vi "GetFileVersion_DotNet.vi"(8 "error in (no error)":errorcluster, 11 "Exe Path":path) -> (0 "error out":errorcluster, 2 "File Info Out":T1, 3 "Exe Path Out":path)   [LabVIEW 2015]
doc: "This VI can obtain information about an existing executable, such as its version, product name, and so on, or it can be called as a subVI from a VI that will be built into an executable to obtain information about that executable.\n\nTo obtain version information about an existing executable, enter a path to an executable into Exe Path and run the Vi.\n\nCall this VI as a subVI from a VI that you will build into an executable and leave the path input unwired to obtain the version information about the built executable."
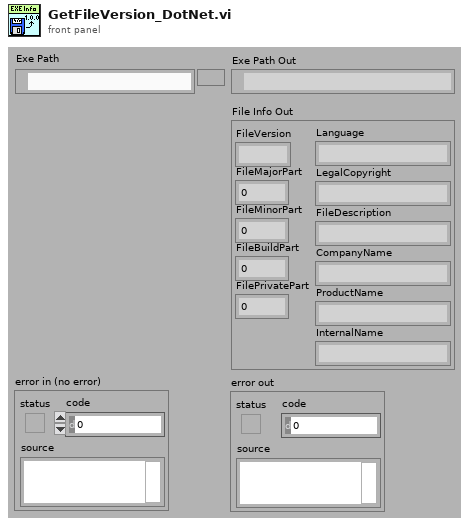
[diagram p1: front panel]
types:
  T1 = cluster{"FileVersion":string, "FileMajorPart":i32, "FileMinorPart":i32, "FileBuildPart":i32, "FilePrivatePart":i32, "Language":string, "LegalCopyright":string, "FileDescription":string, "CompanyName":string, "ProductName":string, "InternalName":string}
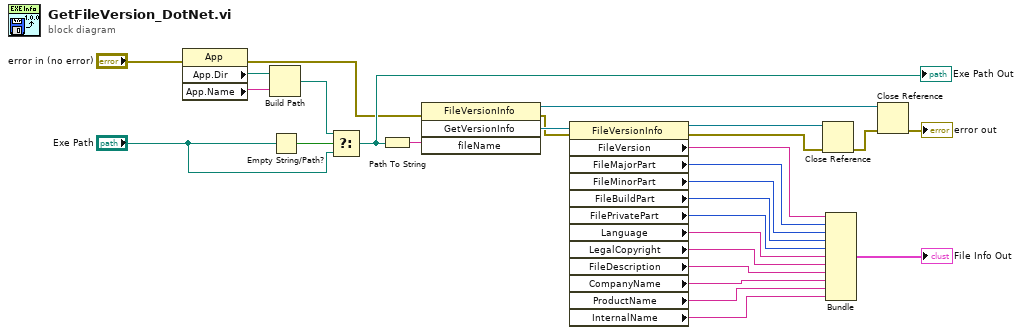
[diagram p0: block diagram]
diagram:
  n1 = property class="App"(error in="error in (no error)") -> (error out=w14:errorcluster, "App.Dir"=w23:path, "App.Name"=w22:string)  [unwired: 1 in, 1 out]
  n2 = Build Path(base path=w23, name or relative path=w22) -> (appended path=w19:path)
  n3 = Empty String/Path?(string/path="Exe Path") -> (empty?=w21:bool)
  n4 = Select(t=w19, s=w21, f="Exe Path") -> (s? t:f=w18:path)
  "Exe Path Out" <- w18
  n5 = Path To String(path=w18) -> (string=w26:string)
  n6 = invoke class="FileVersionInfo" method="GetVersionInfo"(error in=w14, "fileName"=w26) -> (reference out=w15:refnum<k24>, error out=w27:errorcluster, "GetVersionInfo"=w28:refnum<k24>)  [unwired: 2 in, 1 out]
  n7 = property class="FileVersionInfo"(reference=w28, error in=w27) -> (reference out=w25:refnum<k24>, error out=w24:errorcluster, "FileVersion"=w12:string, "FileMajorPart"=w5:i32, "FileMinorPart"=w4:i32, "FileBuildPart"=w11:i32, "FilePrivatePart"=w3:i32, "Language"=w10:string, "LegalCopyright"=w2:string, "FileDescription"=w9:string, "CompanyName"=w1:string, "ProductName"=w8:string, "InternalName"=w7:string)
  n8 = Close Reference(reference=w25, error in (no error)=w24) -> (error out=w16:errorcluster)
  n9 = Bundle("FileVersion"=w12, "FileMajorPart"=w5, "FileMinorPart"=w4, "FileBuildPart"=w11, "FilePrivatePart"=w3, "Language"=w10, "LegalCopyright"=w2, "FileDescription"=w9, "CompanyName"=w1, "ProductName"=w8, "InternalName"=w7) -> (→"File Info Out":T1)  [unwired: 1 in]
  n10 = Close Reference(reference=w15, error in (no error)=w16) -> (error out=→"error out":errorcluster)
